vi "Get_Arr_Dims.vi"(0 "Data":dbl[][](array[numeric])) -> (1 "N Rows":i32, 2 "N Cols":i32, 3 "Valid":bool)   [LabVIEW 2018]
doc: "VI to obtain the dimensions of a 2D matrix\n\nValid == True when Nrows and Ncols both greater than zero\n\nR. Sheehan 2 - 11 - 2017"
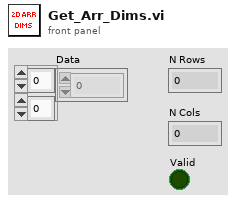
[diagram p1: front panel]
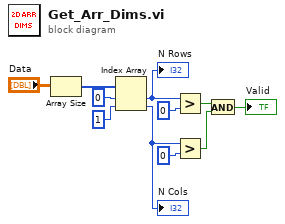
[diagram p0: block diagram]
diagram:
  n1 = Array Size(array="Data") -> (size(s)=w10:i32[])
  n2 = Index Array(array=w10, index #1=0 ("index"), index #2=1 ("index")) -> (element #1=w7:i32, element #2=w4:i32)
  "N Rows" <- w7
  "N Cols" <- w4
  n3 = Greater?(x=w7, y=0) -> (0:w3:bool)
  n4 = Greater?(x=w4, y=0) -> (0:w2:bool)
  n5 = And(x=w3, y=w2) -> (x .and. y?=→"Valid":bool)
